vi "Py_LV.vi"() -> ()   [LabVIEW 2019]
panel:
  out "A+B":i32
  in  "B":i32
  in  "A":i32
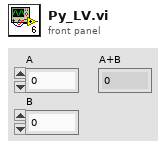
[diagram p1: front panel]
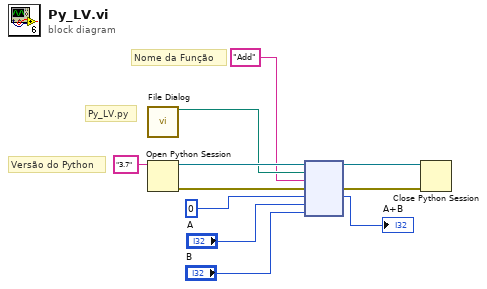
[diagram p0: block diagram]
diagram:
  # "Py_LV.py"
  # "Nome da Função"
  # "Versão do Python"
  n1 = call "File Dialog"() -> ("selected path"=w6:path)  [unwired: 12 in, 3 out]
  n2 = Open Python Session(python version="3.7" ("Python version")) -> (session out=w11:refnum<k35>, error out=w9:errorcluster)  [unwired: 2 in]
  n3 = node(w11, w6, "Add" ("function name"), w9, 0, "A", "B") -> (w10:refnum<k35>, w8:errorcluster, →"A+B":i32)  [unwired: 2 in, 2 out]
  n4 = Close Python Session(session in=w10, error in=w8) -> ()  [unwired: 1 out]
